vi "IMAQ FPGA Pixel Bus to FIFO U8x1.vi"(8 "Input Valid":bool, 10 "Destination Image FIFO":refnum<k21>, 11 "Pixel Bus In":T1) -> (4 "Ready for Input":bool)   [LabVIEW 2020, in "NI_VDM_FPGA_Basics.lvlib"]
doc: "Writes valid Pixel Data in the Pixel Bus cluster to the specified FIFO. If the FIFO is full, the Ready for Input terminal returns FALSE during that cycle."
uses:
  <vilib>/visionFPGA/NI_VDM_FPGA_Basics.lvlib
  <vilib>/rvi/DataTransferAndStorage/Container/XNode/niFpgaContainer.xnode
  <vilib>/rvi/FIFO/Fifo_Resource/niFpgaFifoEmulationRefIn.vi
  <vilib>/visionFPGA/Controls/IMAQ FPGA Pixel Bus u8x1.ctl
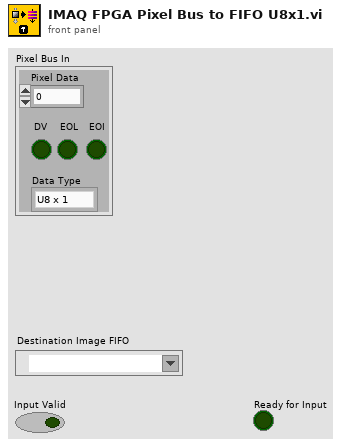
[diagram p1: front panel]
types:
  T1 = typedef "IMAQ FPGA Pixel Bus u8x1.ctl" = cluster{"Pixel Data":u8, "DV":bool, "EOL":bool, "EOI":bool, "Data Type":enum16{"U8 x 1"}}
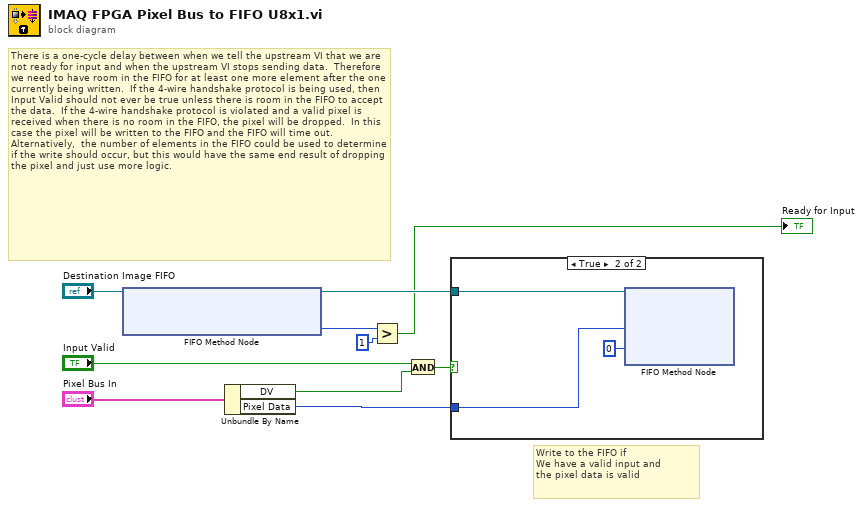
[diagram p0: block diagram]
diagram:
  # "There is a one-cycle delay between when we tell the upstream VI that we are not ready for input and when the upstream VI stops sending data.  Therefore we need to have room in the FIFO for at least one more element after the one currently being written.  If the 4-wire handshake protocol is being used, then Input Valid should not ever be true unless there is room in the FIFO to accept the data.  If the 4-wire handshake protocol is violated and a valid pixel is received when there is no room in the FIFO, the pixel will be dropped.  In this case the pixel will be written to the FIFO and the FIFO will time out.  Alternatively,  the number of elements in the FIFO could be used to determine if the write should occur, but this would have the same end result of dropping the pixel and just use more logic."
  # "Write to the FIFO if \nWe have a valid input and\nthe pixel data is valid"
  n1 = xnode ("FIFO Method Node")("FIFO In"="Destination Image FIFO") -> ("Number of Elements to Write"=w5:u32, "FIFO Out"=w8:refnum<k21>)
  n2 = Unbundle By Name("Pixel Bus In") -> ("DV"=w2:bool, "Pixel Data"=w1:u8)
  n3 = Greater?(x=w5, y=u32 1) -> (0:→"Ready for Input":bool)
  n4 = And(x="Input Valid", y=w2) -> (x .and. y?=w7:bool)
  n5 = case shown="True" w7 {
    tunnel: w8 -> [_ w13]
    tunnel: w1 -> [_ w11]
    frame False {
    }
    frame True {
      n6 = xnode ("FIFO Method Node")("Element"=w11, "Timeout"=0, "FIFO In"=w13) -> ()  [unwired: 2 out]
    }
  }
